vi "Datasheet Plot Styles.vi"(11 "parameters":T1) -> (2 "styles":string[](array[string]), 3 "parameters 2":T1)   [LabVIEW 2011]
uses:
  Addons/internet/utils/keyedarr.llb/Keyed Array.ctl
  Addons/internet/utils/strutil.llb/Case Matching.ctl
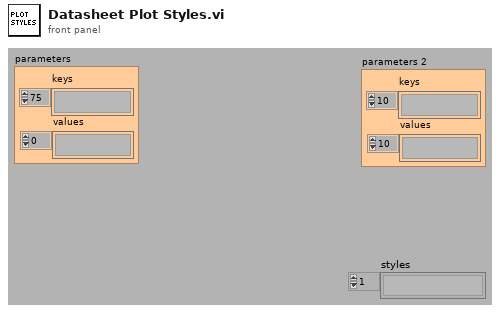
[diagram p1: front panel]
types:
  T1 = typedef "Keyed Array.ctl" = cluster{"keys":string[], "values":string[]}
  T2 = typedef "Case Matching.ctl" = enum16{"a != A", "a == A", "system"}
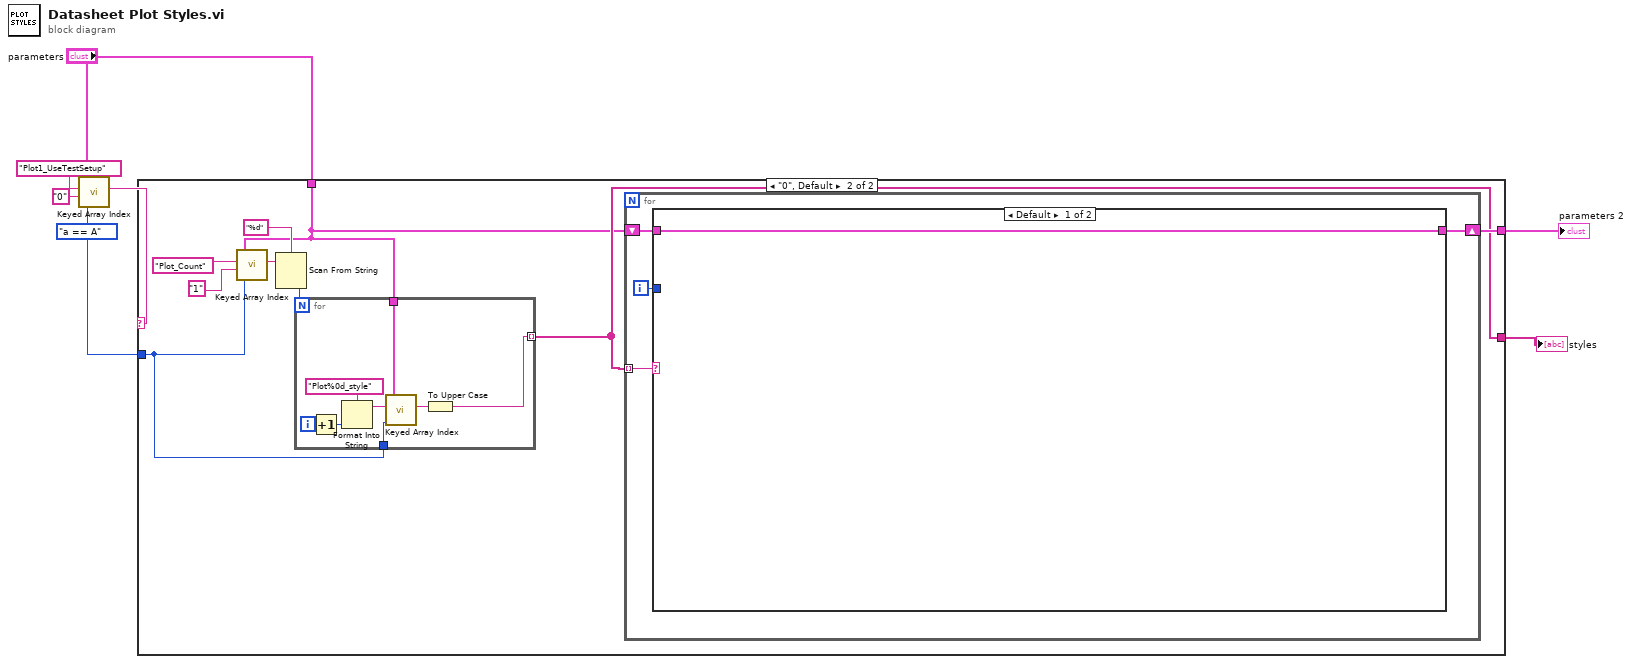
[diagram p0: block diagram]
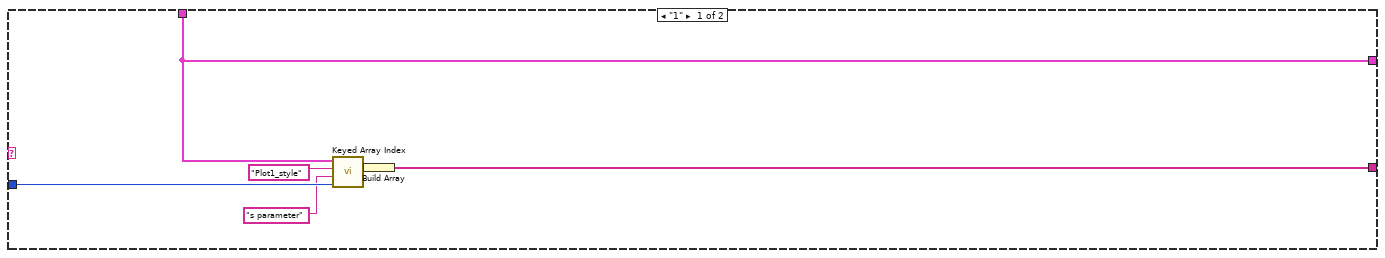
[diagram p2: hidden frame]
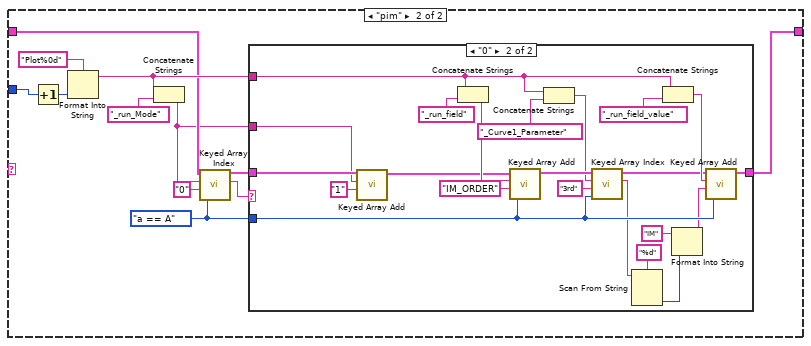
[diagram p3: hidden frame]
diagram:
  w4 = Case_Matching."a == A" ("case matching (sensitive)")
  n1 = call "Keyed Array Index.vi"("case matching (sensitive)"=w4, "default value"="0", "key"="Plot1_UseTestSetup" ("format string"), "array in"="parameters") -> ("value"=w5:string)  [unwired: 3 out]
  n2 = case shown="\"0\", Default" w5 {
    tunnel: [w12 w15] -> w3
    tunnel: "parameters" -> [w8 w14]
    tunnel: w4 -> [w10 w17]
    tunnel: [w8 w16] -> w1
    frame "1" {
      n3 = call "Keyed Array Index.vi"("case matching (sensitive)"=w10, "default value"="s parameter" ("format string"), "key"="Plot1_style" ("format string"), "array in"=w8) -> ("value"=w13:string)  [unwired: 3 out]
      n4 = Build Array(w13) -> (w12:string[])
    }
    frame "0", Default {
      n5 = call "Keyed Array Index.vi"("case matching (sensitive)"=w17, "default value"="1" ("format string"), "key"="Plot_Count" ("format string"), "array in"=w14) -> ("value"=w20:string)  [unwired: 3 out]
      n6 = Scan From String(format string="%d", input string=w20) -> (output 1=w19:i32)  [unwired: 2 in, 4 out]
      n7 = for {
        N: w19 -> [_]
        tunnel: w14 -> [w65]
        tunnel: w17 -> [w64]
        tunnel: [w63] -> w15 mode=indexing
        i -> [w68]
        n8 = Increment(x=w68) -> (x+1=w66:i32)
        n9 = Format Into String(format string="Plot%0d_style", w66) -> (resulting string=w70:string)  [unwired: 2 in, 1 out]
        n10 = call "Keyed Array Index.vi"("case matching (sensitive)"=w64, "key"=w70, "array in"=w65) -> ("value"=w67:string)  [unwired: 1 in, 3 out]
        n11 = To Upper Case(1:w67) -> (0:w63:string)
      }
      n12 = for {
        tunnel: w15 -> [w26] mode=indexing
        shift-right: [w25] -> w16
        shift-left: w14 -> [w24]
        i -> [w23]
        n13 = case shown="Default" w26 {
          tunnel: [w27 w29] -> w25
          tunnel: w24 -> [w27 w31]
          tunnel: w23 -> [_ w33]
          frame Default {
          }
          frame "pim" {
            w34 = Case_Matching."a == A" ("case matching (sensitive)")
            n14 = Increment(x=w33) -> (x+1=w38:i32)
            n15 = Format Into String(format string="Plot%0d", w38) -> (resulting string=w35:string)  [unwired: 2 in, 1 out]
            n16 = Concatenate Strings(w35, "_run_Mode" ("format string")) -> (w28:string)
            n17 = call "Keyed Array Index.vi"("case matching (sensitive)"=w34, "default value"="0", "key"=w28, "array in"=w31) -> ("value"=w30:string, "duplicate array"=w36:T1)  [unwired: 2 out]
            n18 = case shown="\"0\"" w30 {
              tunnel: w36 -> [w40 w43]
              tunnel: w35 -> [_ w52]
              tunnel: w34 -> [_ w54]
              tunnel: [w40 w58] -> w29
              tunnel: w28 -> [_ w41]
              frame Default {
              }
              frame "0" {
                n19 = call "Keyed Array Add.vi"("value"="1", "key"=w41, "array in"=w43) -> ("array out"=w42:T1)  [unwired: 2 in, 2 out]
                n20 = Concatenate Strings(w52, "_run_field" ("format string")) -> (w59:string)
                n21 = call "Keyed Array Add.vi"("case matching (sensitive)"=w54, "value"="IM_ORDER", "key"=w59, "array in"=w42) -> ("array out"=w56:T1)  [unwired: 1 in, 2 out]
                n22 = Concatenate Strings(w52, "_Curve1_Parameter" ("format string")) -> (w51:string)
                n23 = call "Keyed Array Index.vi"("case matching (sensitive)"=w54, "default value"="3rd", "key"=w51, "array in"=w56) -> ("value"=w45:string, "duplicate array"=w55:T1)  [unwired: 2 out]
                n24 = Scan From String(format string="%d", input string=w45) -> (output 1=w48:i32)  [unwired: 3 in, 3 out]
                n25 = Concatenate Strings(w52, "_run_field_value" ("format string")) -> (w60:string)
                n26 = Format Into String(initial string="IM", w48) -> (resulting string=w46:string)  [unwired: 2 in, 1 out]
                n27 = call "Keyed Array Add.vi"("case matching (sensitive)"=w54, "value"=w46, "key"=w60, "array in"=w55) -> ("array out"=w58:T1)  [unwired: 1 in, 2 out]
              }
            }
          }
        }
      }
    }
  }
  "styles" <- w3
  "parameters 2" <- w1
